vi "Write Stop Disk Action.vi"(8 "error in (no error)":errorcluster, 10 "Stop Disk Action":refnum<notifier>, 11 "File Worker in":refnum<class "File Worker.lvclass">) -> (0 "error out":errorcluster, 3 "File Worker out":refnum<class "File Worker.lvclass">)   [LabVIEW 2025, in "File Worker.lvlib" / "File Worker.lvclass"]
uses:
  File Worker.lvclass
  File Worker.lvclass/File Worker.ctl
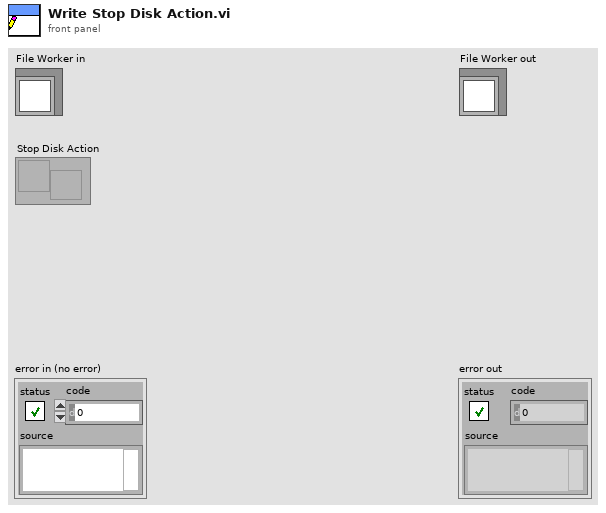
[diagram p1: front panel]
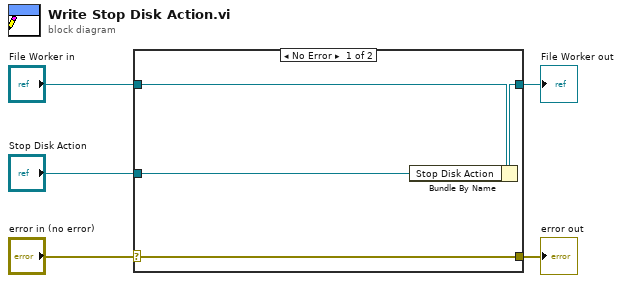
[diagram p0: block diagram]
diagram:
  n1 = case shown="No Error" "error in (no error)" {
    selector: "error in (no error)" -> [w9 w10]
    tunnel: [w9 w10] -> w4
    tunnel: [w7 w11] -> w2
    tunnel: "File Worker in" -> [w8 w11]
    tunnel: "Stop Disk Action" -> [w6 _]
    frame No Error {
      n2 = Bundle By Name(cluster=w8, "Stop Disk Action"=w6) -> (w7:refnum<class "File Worker.lvclass">)
    }
    frame Error {
    }
  }
  "error out" <- w4
  "File Worker out" <- w2
